vi "Variant-Preview.vi"(6 "delimiter (/)":string="/", 8 "error in":errorcluster, 11 "data":variant) -> (0 "error out":errorcluster, 2 "Array":string[][](array[string]), 3 "data(dup)":variant)   [LabVIEW 2019]
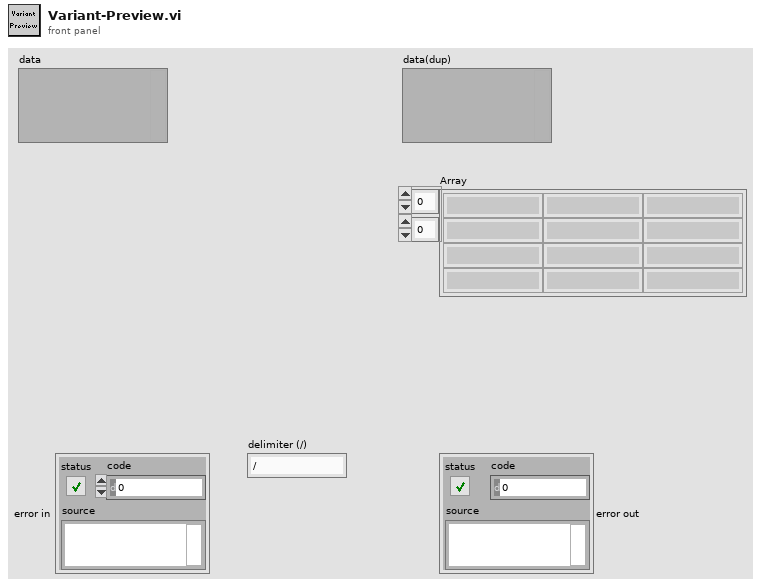
[diagram p1: front panel]
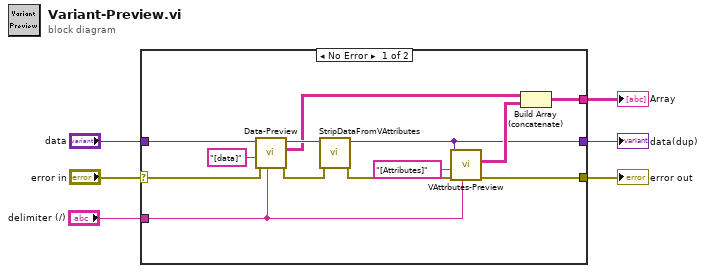
[diagram p0: block diagram]
diagram:
  n1 = case shown="No Error" "error in" {
    selector: "error in" -> [w17 w21]
    tunnel: "data" -> [w18 w20]
    tunnel: [w12 w20] -> w4
    tunnel: [w9 w21] -> w3
    tunnel: [w13 _] -> w2
    tunnel: "delimiter (/)" -> [w16 _]
    frame No Error {
      n2 = call "Data-Preview.vi"("delimiter (/)"=w16, "error in"=w17, "ParentStr"="[data]", "data"=w18) -> ("error out"=w11:errorcluster, "Array"=w15:string[][], "data(dup)"=w19:variant)  [unwired: 5 in]
      n3 = call "StripDataFromVAttributes.vi"("error in (no error)"=w11, "Map"=w19) -> ("error out"=w10:errorcluster, "duplicate variant"=w12:variant)  [unwired: 8 in]
      n4 = call "VAttrbutes-Preview.vi"("delimiter (/)"=w16, "error in"=w10, "ParentStr"="[Attributes]", "VAttributes"=w12) -> ("error out"=w9:errorcluster, "Array"=w14:string[][])  [unwired: 5 in, 1 out]
      n5 = Build Array (concatenate)(w15, w14) -> (w13:string[][])
    }
    frame Error {
    }
  }
  "error out" <- w3
  "data(dup)" <- w4
  "Array" <- w2
